vi "Register Tools Pressed.vi"(8 "error in (no error)":errorcluster, 11 "UI Controller in":refnum<class "UI Controller.lvclass">) -> (0 "error out":errorcluster, 3 "UI Controller out":refnum<class "UI Controller.lvclass">)   [LabVIEW 2020, in "UI Controller.lvlib" / "UI Controller.lvclass"]
uses:
  UI Controller.lvclass
  C:/Program Files/National Instruments/LabVIEW 2020/vi.lib/ActorFrameworkMVC/Abstract Controller/Abstract Controller/Abstract Controller.lvclass
  C:/Program Files/National Instruments/LabVIEW 2020/vi.lib/ActorFramework/Actor/Actor.lvclass
  Views/Menu View/Menu View Messages/Register Tools Pressed Msg/Register Tools Pressed Msg.lvclass
  C:/Program Files/National Instruments/LabVIEW 2020/vi.lib/ActorFramework/Message/Message.lvclass
  UI Controller Messages/Concrete Tools Pressed Msg/Concrete Tools Pressed Msg.lvclass
  C:/Program Files/National Instruments/LabVIEW 2020/vi.lib/ActorFrameworkObserver/Data Message/Data Message.lvclass
  <vilib>/ActorFramework/Actor/Actor.lvclass/Actor.ctl
  <vilib>/ActorFramework/Message Enqueuer/Message Enqueuer.lvclass/Message Enqueuer.ctl
  <vilib>/ActorFramework/Message Enqueuer/Init from Existing Queue.vi
  <vilib>/ActorFramework/Message Priority Queue/Priority Enqueue.vi
  <vilib>/ActorFramework/Message Enqueuer/Message Enqueuer.lvclass
  <vilib>/ActorFrameworkMVC/Abstract Controller/Abstract Controller/Abstract Controller.lvclass
  <vilib>/ActorFramework/Actor/Actor.lvclass
panel:
  # "NOTICE -- YOU MUST LEAVE THIS NOTICE IN PLACE.\n\nCopyright (c) 2017, LIANG LIU Shawn.Liu.cn@gmail.com\nAll rights reserved.\n\nRedistribution and use in source and binary forms, with or without modification, are permitted provided that the following conditions are met:\n-Redistributions of source code must retain the above copyright notice, this list of conditions and the following disclaimer.\n-Redistributions in binary form must reproduce the above copyright notice, this list of conditions and the following disclaimer in the documentation and/or other materials provided with the distribution.\n-Neither the name of the eLp nor the names of its contributors may be used to endorse or promote products derived from this software without specific prior written permission.\n\nTHIS SOFTWARE IS PROVIDED BY THE COPYRIGHT HOLDERS AND CONTRIBUTORS \"AS IS\" AND ANY EXPRESS OR IMPLIED WARRANTIES, INCLUDING, BUT NOT LIMITED TO, THE IMPLIED WARRANTIES OF MERCHANTABILITY AND FITNESS FOR A PARTICULAR PURPOSE ARE DISCLAIMED. IN NO EVENT SHALL THE COPYRIGHT HOLDER OR CONTRIBUTORS BE LIABLE FOR ANY DIRECT, INDIRECT, INCIDENTAL, SPECIAL, EXEMPLARY, OR CONSEQUENTIAL DAMAGES (INCLUDING, BUT NOT LIMITED TO, PROCUREMENT OF SUBSTITUTE GOODS OR SERVICES; LOSS OF USE, DATA, OR PROFITS; OR BUSINESS INTERRUPTION) HOWEVER CAUSED AND ON ANY THEORY OF LIABILITY, WHETHER IN CONTRACT, STRICT LIABILITY, OR TORT (INCLUDING NEGLIGENCE OR OTHERWISE) ARISING IN ANY WAY OUT OF THE USE OF THIS SOFTWARE, EVEN IF ADVISED OF THE POSSIBILITY OF SUCH DAMAGE."
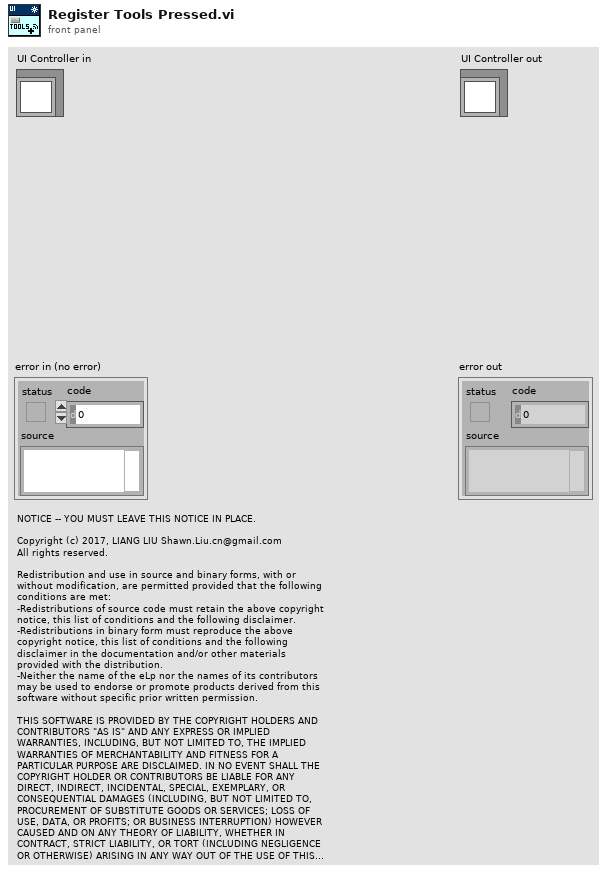
[diagram p1: front panel]
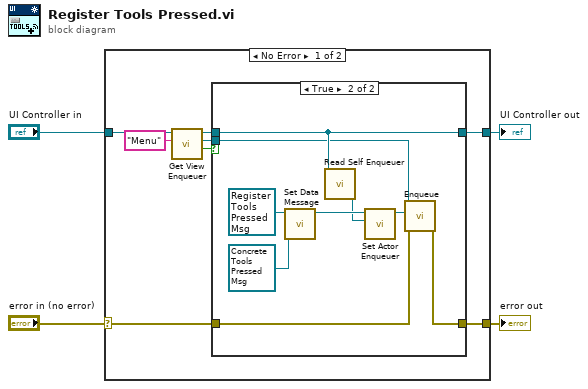
[diagram p0: block diagram]
diagram:
  n1 = case shown="No Error" "error in (no error)" {
    selector: "error in (no error)" -> [w10 w25]
    tunnel: "UI Controller in" -> [w12 w24]
    tunnel: [w11 w24] -> w3
    tunnel: [w9 w25] -> w1
    frame No Error {
      n2 = call <vilib>:"Get View Enqueuer.vi"("View Name"="Menu", "Abstract Controller in"=w12) -> ("Found?"=w7:bool, "View Enqueuer"=w6:refnum<class "Message Enqueuer.lvclass">, "Abstract Controller out"=w5:refnum<class "UI Controller.lvclass">)  [unwired: 6 in, 1 out]
      n3 = case shown="True" w7 {
        tunnel: w6 -> [_ w18]
        tunnel: w5 -> [w14 w19]
        tunnel: [w14 w19] -> w11
        tunnel: w10 -> [w13 w16]
        tunnel: [w13 w15] -> w9
        frame False {
        }
        frame True {
          n4 = call-dynamic "Set Data Message.vi"("Data Message"=refnum<class "Concrete Tools Pressed Msg.lvclass"> refnum ("UI Controller.lvlib:Concrete Tools Pressed Msg.lvclass"), "Registration Message in"=refnum<class "Register Tools Pressed Msg.lvclass"> refnum ("Menu View.lvlib:Register Tools Pressed Msg.lvclass")) -> ("Registration Message out"=w22:refnum<class "Register Tools Pressed Msg.lvclass">)  [unwired: 9 in]
          n5 = call <vilib>:"Read Self Enqueuer.vi"("Actor"=w19) -> ("Self Enqueuer"=w20:refnum<class "Message Enqueuer.lvclass">)  [unwired: 10 in]
          n6 = call-dynamic "Set Actor Enqueuer.vi"("Actor Enqueuer"=w20, "Registration Message in"=w22) -> ("Registration Message out"=w17:refnum<class "Register Tools Pressed Msg.lvclass">)  [unwired: 9 in]
          n7 = call <vilib>:"Enqueue.vi"("error in (no error)"=w16, "Message"=w17, "Message Enqueuer in"=w18) -> ("error out"=w15:errorcluster)  [unwired: 7 in, 1 out]
        }
      }
    }
    frame Error {
    }
  }
  "error out" <- w1
  "UI Controller out" <- w3
